vi "ex7-13.vi"() -> ()   [LabVIEW 2013]
panel:
  out "appended array":dbl[](array[numeric])
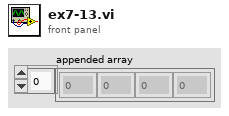
[diagram p1: front panel]
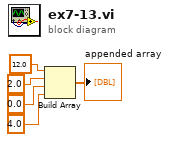
[diagram p0: block diagram]
diagram:
  n1 = Build Array(12.0 ("element"), 2.0 ("element"), 0.0 ("element"), 4.0 ("element")) -> (→"appended array":dbl[])
